vi "stop_DAQmxTasks.vi"(8 "error in (no error)":errorcluster, 11 "cluster of DAQ tasks":T1) -> (0 "error out":errorcluster)   [LabVIEW 2015]
uses:
  controls/Daqmxtasks.ctl
  <vilib>/DAQmx/write.llb/DAQmx Write (Digital Bool 1Line 1Point).vi
  <vilib>/DAQmx/miscellaneous.llb/DAQmx Fill In Error Info.vi
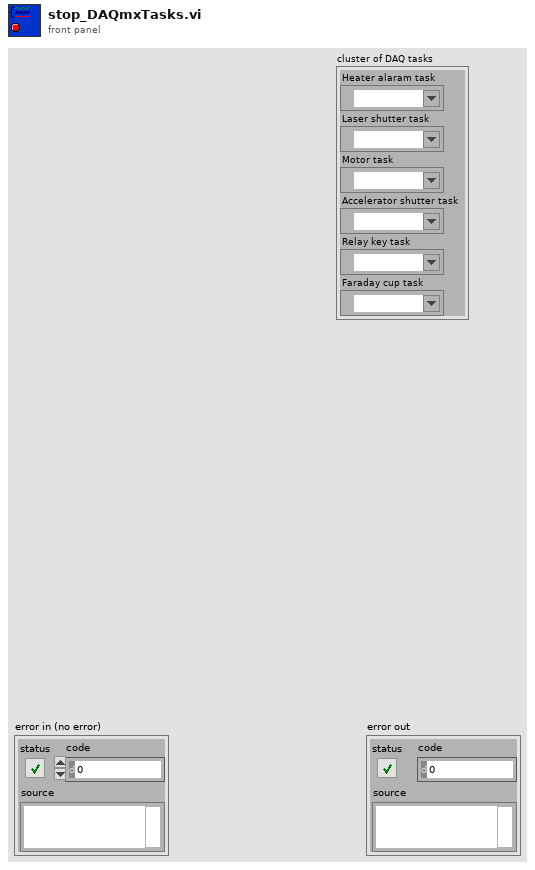
[diagram p1: front panel]
types:
  T1 = typedef "Daqmxtasks.ctl" = cluster{"Heater alaram task":refnum<k21>, "Laser shutter task":refnum<k21>, "Motor task":refnum<k21>, "Accelerator shutter task":refnum<k21>, "Relay key task":refnum<k21>, "Faraday cup task":refnum<k21>}
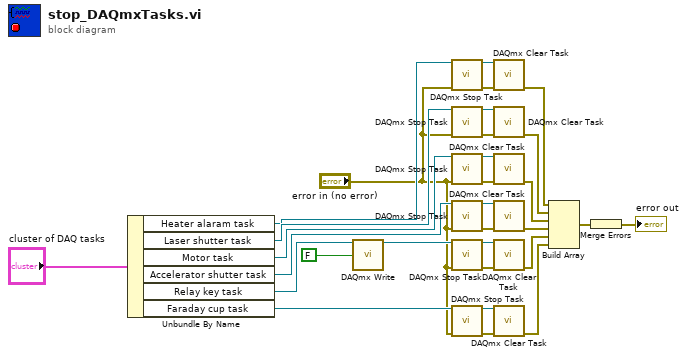
[diagram p0: block diagram]
diagram:
  n1 = Unbundle By Name("cluster of DAQ tasks") -> ("Heater alaram task"=w27:refnum<k21>, "Laser shutter task"=w28:refnum<k21>, "Motor task"=w29:refnum<k21>, "Accelerator shutter task"=w30:refnum<k21>, "Relay key task"=w26:refnum<k21>, "Faraday cup task"=w4:refnum<k21>)
  n2 = call-poly <vilib>:"DAQmx Write.vi"("task/channels in"=w26, "data"=FALSE) -> ("task out"=w24:refnum<k21>)  [unwired: 11 in, 2 out]
  n3 = call <vilib>:"DAQmx Stop Task.vi"("task/channels in"=w27, "error in"="error in (no error)") -> ("task out"=w12:refnum<k21>, "error out"=w13:errorcluster)  [unwired: 12 in]
  n4 = call <vilib>:"DAQmx Stop Task.vi"("task/channels in"=w28, "error in"="error in (no error)") -> ("task out"=w11:refnum<k21>, "error out"=w7:errorcluster)  [unwired: 12 in]
  n5 = call <vilib>:"DAQmx Stop Task.vi"("task/channels in"=w29, "error in"="error in (no error)") -> ("task out"=w10:refnum<k21>, "error out"=w14:errorcluster)  [unwired: 12 in]
  n6 = call <vilib>:"DAQmx Stop Task.vi"("task/channels in"=w30, "error in"="error in (no error)") -> ("task out"=w9:refnum<k21>, "error out"=w8:errorcluster)  [unwired: 12 in]
  n7 = call <vilib>:"DAQmx Stop Task.vi"("task/channels in"=w24, "error in"="error in (no error)") -> ("task out"=w22:refnum<k21>, "error out"=w21:errorcluster)  [unwired: 12 in]
  n8 = call <vilib>:"DAQmx Stop Task.vi"("task/channels in"=w4, "error in"="error in (no error)") -> ("task out"=w2:refnum<k21>, "error out"=w5:errorcluster)  [unwired: 12 in]
  n9 = call <vilib>:"DAQmx Clear Task.vi"("task in"=w12, "error in"=w13) -> ("error out"=w15:errorcluster)  [unwired: 13 in]
  n10 = call <vilib>:"DAQmx Clear Task.vi"("task in"=w11, "error in"=w7) -> ("error out"=w16:errorcluster)  [unwired: 13 in]
  n11 = call <vilib>:"DAQmx Clear Task.vi"("task in"=w10, "error in"=w14) -> ("error out"=w17:errorcluster)  [unwired: 13 in]
  n12 = call <vilib>:"DAQmx Clear Task.vi"("task in"=w9, "error in"=w8) -> ("error out"=w18:errorcluster)  [unwired: 13 in]
  n13 = call <vilib>:"DAQmx Clear Task.vi"("task in"=w22, "error in"=w21) -> ("error out"=w23:errorcluster)  [unwired: 13 in]
  n14 = call <vilib>:"DAQmx Clear Task.vi"("task in"=w2, "error in"=w5) -> ("error out"=w1:errorcluster)  [unwired: 13 in]
  n15 = Build Array(w15, w16, w17, w18, w23, w1) -> (w19:errorcluster[])
  n16 = Merge Errors(w19) -> (→"error out":errorcluster)
